vi "GT Get Trap Prm.vi"(8 "error in (no error)":errorcluster caption="错误输入（无错误）", 9 "pPrm":T1, 10 "profile":i16, 11 "cardNum":i16) -> (0 "error out":errorcluster caption="错误输出", 1 "pPrm out":T1, 3 "function return":i16)   [LabVIEW 2014, in "gts.lvlib"]
doc: "GT_API GT_GetTrapPrm(short cardNum,short profile,TTrapPrm *pPrm);"
uses:
  gts.lvlib
  gts.dll
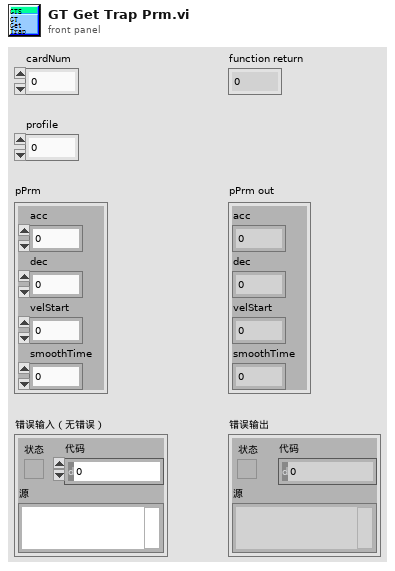
[diagram p1: front panel]
types:
  T1 = cluster{"acc":dbl, "dec":dbl, "velStart":dbl, "smoothTime":i16}
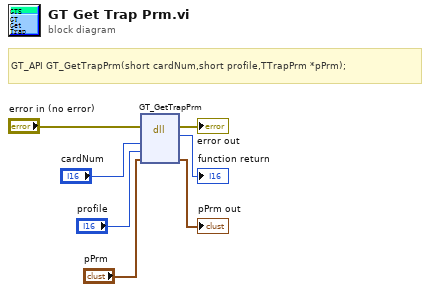
[diagram p0: block diagram]
diagram:
  # "GT_API GT_GetTrapPrm(short cardNum,short profile,TTrapPrm *pPrm);"
  n1 = dll-call lib="PTH2>abs F.多卡库-控制卡基本运动例程(labview)gts.*" fn="GT_GetTrapPrm"(error in="error in (no error)", "cardNum"="cardNum", "profile"="profile", "pPrm"="pPrm") -> (error out=→"error out":errorcluster, →"function return":i16, "pPrm"=→"pPrm out":T1)  [unwired: 4 in, 1 out]
